vi "sub_ctrref_fgv.vi"(7 "cmd":enum16{"write", "read"}(ring), 11 "ctr_in":T1) -> (3 "ctr_out":T1)   [LabVIEW 2018]
uses:
  ctl/ctr-ref.ctl
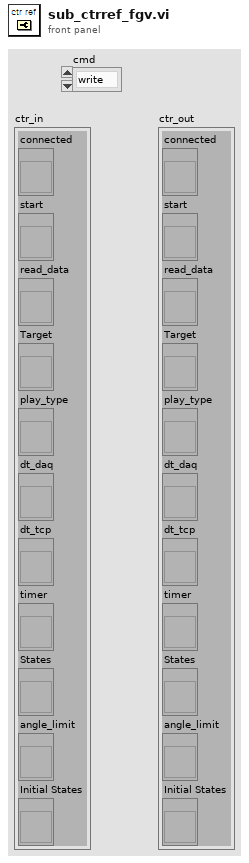
[diagram p1: front panel]
types:
  T1 = typedef "ctr-ref.ctl" = cluster{"connected":refnum<vi>, "start":refnum<vi>, "read_data":refnum<vi>, "Target":refnum<vi>, "play_type":refnum<vi>, "dt_daq":refnum<vi>, "dt_tcp":refnum<vi>, "timer":refnum<vi>, "States":refnum<vi>, "angle_limit":refnum<vi>, "Initial States":refnum<vi>}
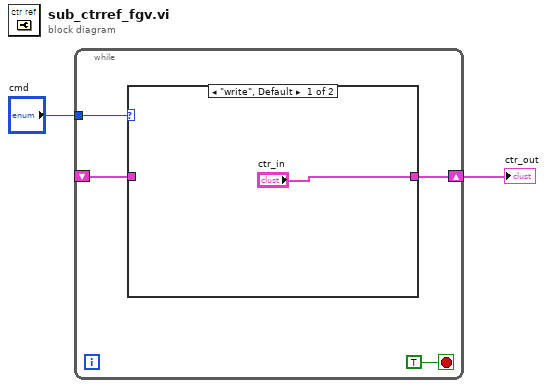
[diagram p0: block diagram]
diagram:
  n1 = while {
    tunnel: "cmd" -> [w5]
    shift-right: [w4] -> w1
    shift-left: _ -> [w3]
    stop <- TRUE stop-if-true
    n2 = case shown="\"write\", Default" w5 {
      tunnel: ["ctr_in" w8] -> w4
      tunnel: w3 -> [_ w8]
      frame "write", Default {
      }
      frame "read" {
      }
    }
  }
  "ctr_out" <- w1
